vi "Analog Output User Interface.vi"() -> ()   [LabVIEW 2023, in "GUI.lvlib" / "Diagnostic.lvlib"]
uses:
  Diagnostic.lvlib
  Control/Analog Output 6739.ctl
  Control/Analog Output.ctl
  Control/Analog Output 6738.ctl
  HardwareAbstractionLayer_LVOOP/Analog Output/NI Analog Output/NI Analog Output.lvclass
  D:/eDCU LTT/VT LTT Project/Source Code/HardwareAbstractionLayer_LVOOP/Analog Output/AO/AO.lvclass
  HardwareAbstractionLayer_LVOOP/Database/SQL Public VI/Control/DB Options.ctl
  HardwareAbstractionLayer_LVOOP/Main/Class Ref.ctl
  HardwareAbstractionLayer_LVOOP/DMM/DMM.lvclass
  HardwareAbstractionLayer_LVOOP/Function Generator/Function Generator.lvclass
  HardwareAbstractionLayer_LVOOP/Oscilloscope/Oscilloscope.lvclass
  HardwareAbstractionLayer_LVOOP/PowerSupply/PowerSupply.lvclass
  HardwareAbstractionLayer_LVOOP/Teststand/Teststand.lvclass
  HardwareAbstractionLayer_LVOOP/Analog Output/AO/AO.lvclass
  HardwareAbstractionLayer_LVOOP/Analog Input/AI/AI.lvclass
  HardwareAbstractionLayer_LVOOP/Database/Database.lvclass
  HardwareAbstractionLayer_LVOOP/Digital Output/DO_class/DO.lvclass
  HardwareAbstractionLayer_LVOOP/Digital Input/DI_class/DI.lvclass
  HardwareAbstractionLayer_LVOOP/PWM Output/PWM Output_class/PWM Output.lvclass
  HardwareAbstractionLayer_LVOOP/PWM Input/PWM Input_class/PWM Input.lvclass
  HardwareAbstractionLayer_LVOOP/NI Switch/NISwitch_class/NISwitch.lvclass
  HardwareAbstractionLayer_LVOOP/Modbus/Modbus_class/Modbus.lvclass
  HardwareAbstractionLayer_LVOOP/CAN/CAN Lib/CAN_class/CAN.lvclass
  HardwareAbstractionLayer_LVOOP/Main/Main.lvclass
panel:
  in  "Stop Acquire":bool
  in  "Start Acquire":bool
  out "error out":errorcluster
  in  "error in":errorcluster
  in  "Operation":T1(tab)
  in  "PXIe - 6739 M1":T2 {"Channel 63" min=-10.0 max=10.0 step=0.1 format="%#.2g"; "Channel 62" min=-10.0 max=10.0 step=0.1 format="%#.2g"; "Channel 61" min=-10.0 max=10.0 step=0.1 format="%#.2g"; "Channel 60" min=-10.0 max=10.0 step=0.1 format="%#.2g"; "Channel 59" min=-10.0 max=10.0 step=0.1 format="%#.2g"; "Channel 58" min=-10.0 max=10.0 step=0.1 format="%#.2g"; "Channel 57" min=-10.0 max=10.0 step=0.1 format="%#.2g"; "Channel 56" min=-10.0 max=10.0 step=0.1 format="%#.2g"; "Channel 55" min=-10.0 max=10.0 step=0.1 format="%#.2g"; "Channel 54" min=-10.0 max=10.0 step=0.1 format="%#.2g"; "Channel 53" min=-10.0 max=10.0 step=0.1 format="%#.2g"; "Channel 52" min=-10.0 max=10.0 step=0.1 format="%#.2g"; "Channel 51" min=-10.0 max=10.0 step=0.1 format="%#.2g"; "Channel 50" min=-10.0 max=10.0 step=0.1 format="%#.2g"; "Channel 49" min=-10.0 max=10.0 step=0.1 format="%#.2g"; "Channel 48" min=-10.0 max=10.0 step=0.1 format="%#.2g"; "Channel 47" min=-10.0 max=10.0 step=0.1 format="%#.2g"; "Channel 46" min=-10.0 max=10.0 step=0.1 format="%#.2g"; "Channel 45" min=-10.0 max=10.0 step=0.1 format="%#.2g"; "Channel 44" min=-10.0 max=10.0 step=0.1 format="%#.2g"; "Channel 43" min=-10.0 max=10.0 step=0.1 format="%#.2g"; "Channel 42" min=-10.0 max=10.0 step=0.1 format="%#.2g"; "Channel 41" min=-10.0 max=10.0 step=0.1 format="%#.2g"; "Channel 40" min=-10.0 max=10.0 step=0.1 format="%#.2g"; "Channel 39" min=-10.0 max=10.0 step=0.1 format="%#.2g"; "Channel 38" min=-10.0 max=10.0 step=0.1 format="%#.2g"; "Channel 37" min=-10.0 max=10.0 step=0.1 format="%#.2g"; "Channel 36" min=-10.0 max=10.0 step=0.1 format="%#.2g"; "Channel 35" min=-10.0 max=10.0 step=0.1 format="%#.2g"; "Channel 34" min=-10.0 max=10.0 step=0.1 format="%#.2g"; "Channel 33" min=-10.0 max=10.0 step=0.1 format="%#.2g"; "Channel 32" min=-10.0 max=10.0 step=0.1 format="%#.2g"; "Channel 31" min=-10.0 max=10.0 step=0.1 format="%#.2g"; "Channel 30" min=-10.0 max=10.0 step=0.1 format="%#.2g"; "Channel 29" min=-10.0 max=10.0 step=0.1 format="%#.2g"; "Channel 28" min=-10.0 max=10.0 step=0.1 format="%#.2g"; "Channel 27" min=-10.0 max=10.0 step=0.1 format="%#.2g"; "Channel 26" min=-10.0 max=10.0 step=0.1 format="%#.2g"; "Channel 25" min=-10.0 max=10.0 step=0.1 format="%#.2g"; "Channel 24" min=-10.0 max=10.0 step=0.1 format="%#.2g"; "Channel 23" min=-10.0 max=10.0 step=0.1 format="%#.2g"; "Channel 22" min=-10.0 max=10.0 step=0.1 format="%#.2g"; "Channel 21" min=-10.0 max=10.0 step=0.1 format="%#.2g"; "Channel 20" min=-10.0 max=10.0 step=0.1 format="%#.2g"; "Channel 19" min=-10.0 max=10.0 step=0.1 format="%#.2g"; "Channel 18" min=-10.0 max=10.0 step=0.1 format="%#.2g"; "Channel 17" min=-10.0 max=10.0 step=0.1 format="%#.2g"; "Channel 16" min=-10.0 max=10.0 step=0.1 format="%#.2g"; "Channel 15" min=-10.0 max=10.0 step=0.1 format="%#.2g"; "Channel 14" min=-10.0 max=10.0 step=0.1 format="%#.2g"; "Channel 13" min=-10.0 max=10.0 step=0.1 format="%#.2g"; "Channel 12" min=-10.0 max=10.0 step=0.1 format="%#.2g"; "Channel 11" min=-10.0 max=10.0 step=0.1 format="%#.2g"; "Channel 10" min=-10.0 max=10.0 step=0.1 format="%#.2g"; "Channel 9" min=-10.0 max=10.0 step=0.1 format="%#.2g"; "Channel 8" min=-10.0 max=10.0 step=0.1 format="%#.2g"; "Channel 7" min=-10.0 max=10.0 step=0.1 format="%#.2g"; "Channel 6" min=-10.0 max=10.0 step=0.1 format="%#.2g"; "Channel 5" min=-10.0 max=10.0 step=0.1 format="%#.2g"; "Channel 4" min=-10.0 max=10.0 step=0.1 format="%#.2g"; "Channel 3" min=-10.0 max=10.0 step=0.1 format="%#.2g"; "Channel 2" min=-10.0 max=10.0 step=0.1 format="%#.2g"; "Channel 1" min=-10.0 max=10.0 step=0.1 format="%#.2g"; "Channel 0" min=-10.0 max=10.0 step=0.1 format="%#.2g"}
  in  "PXIe - 6739 M2":T2 {"Channel 63" min=-10.0 max=10.0 step=0.1 format="%#.2g"; "Channel 62" min=-10.0 max=10.0 step=0.1 format="%#.2g"; "Channel 61" min=-10.0 max=10.0 step=0.1 format="%#.2g"; "Channel 60" min=-10.0 max=10.0 step=0.1 format="%#.2g"; "Channel 59" min=-10.0 max=10.0 step=0.1 format="%#.2g"; "Channel 58" min=-10.0 max=10.0 step=0.1 format="%#.2g"; "Channel 57" min=-10.0 max=10.0 step=0.1 format="%#.2g"; "Channel 56" min=-10.0 max=10.0 step=0.1 format="%#.2g"; "Channel 55" min=-10.0 max=10.0 step=0.1 format="%#.2g"; "Channel 54" min=-10.0 max=10.0 step=0.1 format="%#.2g"; "Channel 53" min=-10.0 max=10.0 step=0.1 format="%#.2g"; "Channel 52" min=-10.0 max=10.0 step=0.1 format="%#.2g"; "Channel 51" min=-10.0 max=10.0 step=0.1 format="%#.2g"; "Channel 50" min=-10.0 max=10.0 step=0.1 format="%#.2g"; "Channel 49" min=-10.0 max=10.0 step=0.1 format="%#.2g"; "Channel 48" min=-10.0 max=10.0 step=0.1 format="%#.2g"; "Channel 47" min=-10.0 max=10.0 step=0.1 format="%#.2g"; "Channel 46" min=-10.0 max=10.0 step=0.1 format="%#.2g"; "Channel 45" min=-10.0 max=10.0 step=0.1 format="%#.2g"; "Channel 44" min=-10.0 max=10.0 step=0.1 format="%#.2g"; "Channel 43" min=-10.0 max=10.0 step=0.1 format="%#.2g"; "Channel 42" min=-10.0 max=10.0 step=0.1 format="%#.2g"; "Channel 41" min=-10.0 max=10.0 step=0.1 format="%#.2g"; "Channel 40" min=-10.0 max=10.0 step=0.1 format="%#.2g"; "Channel 39" min=-10.0 max=10.0 step=0.1 format="%#.2g"; "Channel 38" min=-10.0 max=10.0 step=0.1 format="%#.2g"; "Channel 37" min=-10.0 max=10.0 step=0.1 format="%#.2g"; "Channel 36" min=-10.0 max=10.0 step=0.1 format="%#.2g"; "Channel 35" min=-10.0 max=10.0 step=0.1 format="%#.2g"; "Channel 34" min=-10.0 max=10.0 step=0.1 format="%#.2g"; "Channel 33" min=-10.0 max=10.0 step=0.1 format="%#.2g"; "Channel 32" min=-10.0 max=10.0 step=0.1 format="%#.2g"; "Channel 31" min=-10.0 max=10.0 step=0.1 format="%#.2g"; "Channel 30" min=-10.0 max=10.0 step=0.1 format="%#.2g"; "Channel 29" min=-10.0 max=10.0 step=0.1 format="%#.2g"; "Channel 28" min=-10.0 max=10.0 step=0.1 format="%#.2g"; "Channel 27" min=-10.0 max=10.0 step=0.1 format="%#.2g"; "Channel 26" min=-10.0 max=10.0 step=0.1 format="%#.2g"; "Channel 25" min=-10.0 max=10.0 step=0.1 format="%#.2g"; "Channel 24" min=-10.0 max=10.0 step=0.1 format="%#.2g"; "Channel 23" min=-10.0 max=10.0 step=0.1 format="%#.2g"; "Channel 22" min=-10.0 max=10.0 step=0.1 format="%#.2g"; "Channel 21" min=-10.0 max=10.0 step=0.1 format="%#.2g"; "Channel 20" min=-10.0 max=10.0 step=0.1 format="%#.2g"; "Channel 19" min=-10.0 max=10.0 step=0.1 format="%#.2g"; "Channel 18" min=-10.0 max=10.0 step=0.1 format="%#.2g"; "Channel 17" min=-10.0 max=10.0 step=0.1 format="%#.2g"; "Channel 16" min=-10.0 max=10.0 step=0.1 format="%#.2g"; "Channel 15" min=-10.0 max=10.0 step=0.1 format="%#.2g"; "Channel 14" min=-10.0 max=10.0 step=0.1 format="%#.2g"; "Channel 13" min=-10.0 max=10.0 step=0.1 format="%#.2g"; "Channel 12" min=-10.0 max=10.0 step=0.1 format="%#.2g"; "Channel 11" min=-10.0 max=10.0 step=0.1 format="%#.2g"; "Channel 10" min=-10.0 max=10.0 step=0.1 format="%#.2g"; "Channel 9" min=-10.0 max=10.0 step=0.1 format="%#.2g"; "Channel 8" min=-10.0 max=10.0 step=0.1 format="%#.2g"; "Channel 7" min=-10.0 max=10.0 step=0.1 format="%#.2g"; "Channel 6" min=-10.0 max=10.0 step=0.1 format="%#.2g"; "Channel 5" min=-10.0 max=10.0 step=0.1 format="%#.2g"; "Channel 4" min=-10.0 max=10.0 step=0.1 format="%#.2g"; "Channel 3" min=-10.0 max=10.0 step=0.1 format="%#.2g"; "Channel 2" min=-10.0 max=10.0 step=0.1 format="%#.2g"; "Channel 1" min=-10.0 max=10.0 step=0.1 format="%#.2g"; "Channel 0" min=-10.0 max=10.0 step=0.1 format="%#.2g"}
  in  "PXIe - 6738 M1":T4 {"Channel 31" min=-10.0 max=10.0 step=0.1 format="%#.2g"; "Channel 30" min=-10.0 max=10.0 step=0.1 format="%#.2g"; "Channel 29" min=-10.0 max=10.0 step=0.1 format="%#.2g"; "Channel 28" min=-10.0 max=10.0 step=0.1 format="%#.2g"; "Channel 27" min=-10.0 max=10.0 step=0.1 format="%#.2g"; "Channel 26" min=-10.0 max=10.0 step=0.1 format="%#.2g"; "Channel 25" min=-10.0 max=10.0 step=0.1 format="%#.2g"; "Channel 24" min=-10.0 max=10.0 step=0.1 format="%#.2g"; "Channel 23" min=-10.0 max=10.0 step=0.1 format="%#.2g"; "Channel 22" min=-10.0 max=10.0 step=0.1 format="%#.2g"; "Channel 21" min=-10.0 max=10.0 step=0.1 format="%#.2g"; "Channel 20" min=-10.0 max=10.0 step=0.1 format="%#.2g"; "Channel 19" min=-10.0 max=10.0 step=0.1 format="%#.2g"; "Channel 18" min=-10.0 max=10.0 step=0.1 format="%#.2g"; "Channel 17" min=-10.0 max=10.0 step=0.1 format="%#.2g"; "Channel 16" min=-10.0 max=10.0 step=0.1 format="%#.2g"; "Channel 15" min=-10.0 max=10.0 step=0.1 format="%#.2g"; "Channel 14" min=-10.0 max=10.0 step=0.1 format="%#.2g"; "Channel 13" min=-10.0 max=10.0 step=0.1 format="%#.2g"; "Channel 12" min=-10.0 max=10.0 step=0.1 format="%#.2g"; "Channel 11" min=-10.0 max=10.0 step=0.1 format="%#.2g"; "Channel 10" min=-10.0 max=10.0 step=0.1 format="%#.2g"; "Channel 9" min=-10.0 max=10.0 step=0.1 format="%#.2g"; "Channel 8" min=-10.0 max=10.0 step=0.1 format="%#.2g"; "Channel 7" min=-10.0 max=10.0 step=0.1 format="%#.2g"; "Channel 6" min=-10.0 max=10.0 step=0.1 format="%#.2g"; "Channel 5" min=-10.0 max=10.0 step=0.1 format="%#.2g"; "Channel 4" min=-10.0 max=10.0 step=0.1 format="%#.2g"; "Channel 3" min=-10.0 max=10.0 step=0.1 format="%#.2g"; "Channel 2" min=-10.0 max=10.0 step=0.1 format="%#.2g"; "Channel 1" min=-10.0 max=10.0 step=0.1 format="%#.2g"; "Channel 0" min=-10.0 max=10.0 step=0.1 format="%#.2g"}
  in  "Stop":bool caption="Blank"
  in  "Write":bool caption="Blank"
  # "Analog Output"
  # "Device:"
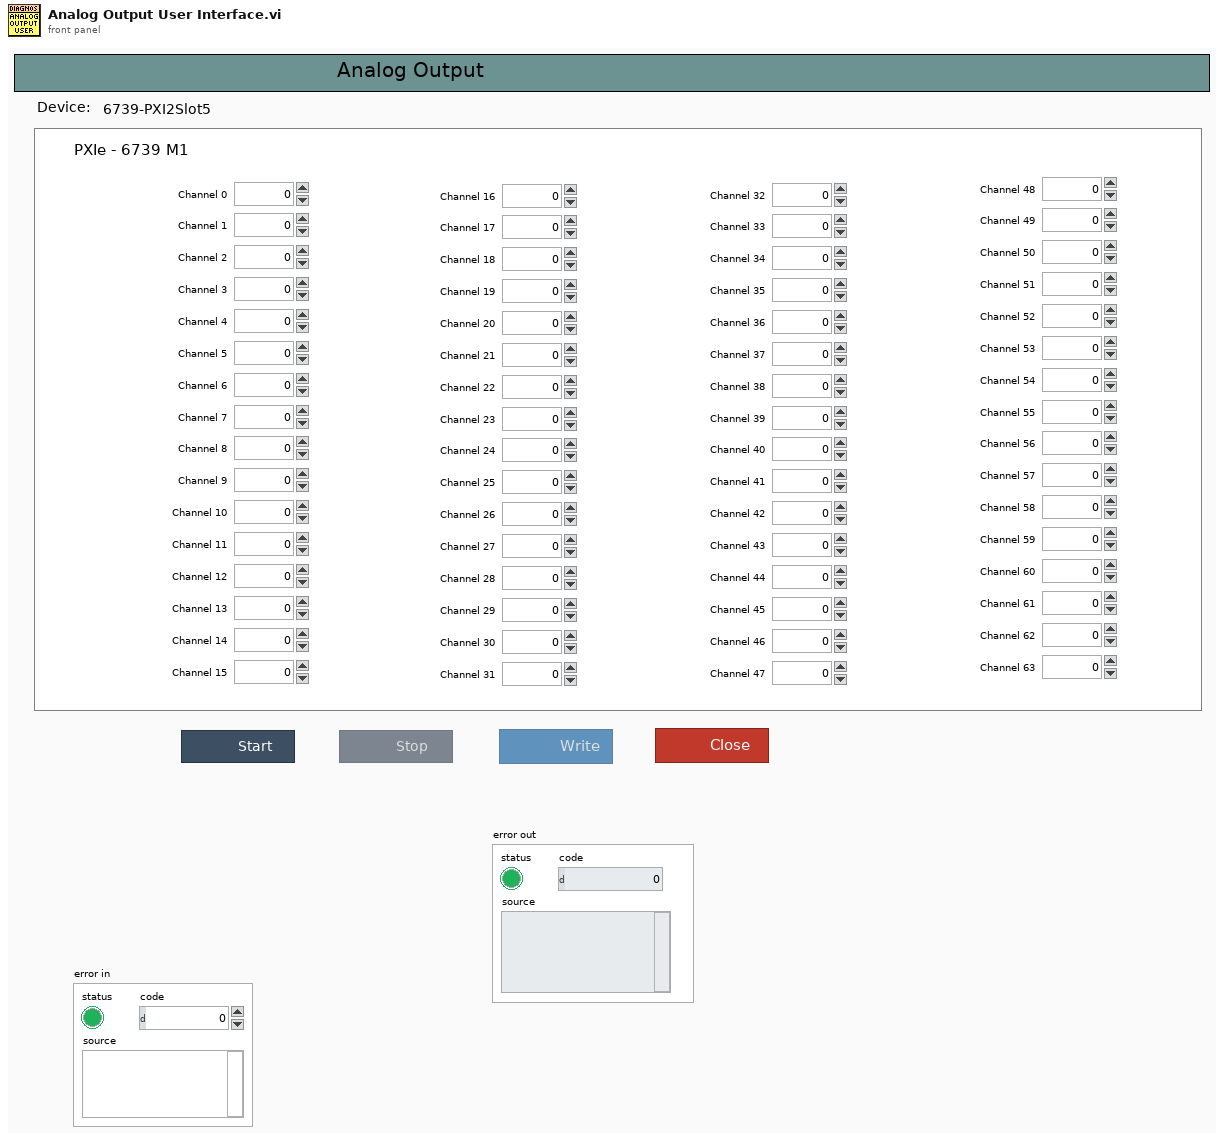
[diagram p1: front panel]
types:
  T1 = enum32{"6739-PXI2Slot5", "6739-PXI2Slot6", "6738-PXI2Slot4"}
  T2 = typedef "GUI.lvlib/Diagnostic.lvlib/Analog Output 6739.ctl" = cluster{"Channel 0":T3, "Channel 1":T3, "Channel 2":T3, "Channel 3":T3, "Channel 4":T3, "Channel 5":T3, "Channel 6":T3, "Channel 7":T3, "Channel 8":T3, "Channel 9":T3, "Channel 10":T3, "Channel 11":T3, "Channel 12":T3, "Channel 13":T3, "Channel 14":T3, "Channel 15":T3, "Channel 16":T3, "Channel 17":T3, "Channel 18":T3, "Channel 19":T3, "Channel 20":T3, "Channel 21":T3, "Channel 22":T3, "Channel 23":T3, "Channel 24":T3, "Channel 25":T3, "Channel 26":T3, "Channel 27":T3, "Channel 28":T3, "Channel 29":T3, "Channel 30":T3, "Channel 31":T3, "Channel 32":T3, "Channel 33":T3, "Channel 34":T3, "Channel 35":T3, "Channel 36":T3, "Channel 37":T3, "Channel 38":T3, "Channel 39":T3, "Channel 40":T3, "Channel 41":T3, "Channel 42":T3, "Channel 43":T3, "Channel 44":T3, "Channel 45":T3, "Channel 46":T3, "Channel 47":T3, "Channel 48":T3, "Channel 49":T3, "Channel 50":T3, "Channel 51":T3, "Channel 52":T3, "Channel 53":T3, "Channel 54":T3, "Channel 55":T3, "Channel 56":T3, "Channel 57":T3, "Channel 58":T3, "Channel 59":T3, "Channel 60":T3, "Channel 61":T3, "Channel 62":T3, "Channel 63":T3}
  T3 = typedef "GUI.lvlib/Diagnostic.lvlib/Analog Output.ctl" = dbl
  T4 = typedef "GUI.lvlib/Diagnostic.lvlib/Analog Output 6738.ctl" = cluster{"Channel 0":T3, "Channel 1":T3, "Channel 2":T3, "Channel 3":T3, "Channel 4":T3, "Channel 5":T3, "Channel 6":T3, "Channel 7":T3, "Channel 8":T3, "Channel 9":T3, "Channel 10":T3, "Channel 11":T3, "Channel 12":T3, "Channel 13":T3, "Channel 14":T3, "Channel 15":T3, "Channel 16":T3, "Channel 17":T3, "Channel 18":T3, "Channel 19":T3, "Channel 20":T3, "Channel 21":T3, "Channel 22":T3, "Channel 23":T3, "Channel 24":T3, "Channel 25":T3, "Channel 26":T3, "Channel 27":T3, "Channel 28":T3, "Channel 29":T3, "Channel 30":T3, "Channel 31":T3}
  T5 = typedef "HardwareAbstractionLayer_LVOOP.lvlib/Database.lvclass/DB Options.ctl" = enum16{"Init", "Select Data", "Insert Data", "Update Data", "Delete Data", "Execute Query", "Create Schema", "Create Table", "List Tables", "List Columns", "Close"}
  T6 = typedef "HardwareAbstractionLayer_LVOOP.lvlib/Main.lvclass/Class Ref.ctl" = cluster{"DMM":refnum<class "DMM.lvclass">, "Function Generator":refnum<class "Function Generator.lvclass">, "Oscilloscope":refnum<class "Oscilloscope.lvclass">, "PowerSupply":refnum<class "PowerSupply.lvclass">, "Teststand":refnum<class "Teststand.lvclass">, "AO":refnum<class "AO.lvclass">, "AI":refnum<class "AI.lvclass">, "Database":refnum<class "Database.lvclass">, "AO Waveform Generation":refnum<class "AO.lvclass">, "DO":refnum<class "DO.lvclass">, "DI":refnum<class "DI.lvclass">, "PWM Output":refnum<class "PWM Output.lvclass">, "PWM Input":refnum<class "PWM Input.lvclass">, "RelayOutput":refnum<class "NISwitch.lvclass">, "Modbus":refnum<class "Modbus.lvclass">, "CAN":refnum<class "CAN.lvclass">}
  T7 = enum8{"Enabled", "Disabled", "Disabled and Grayed Out"}
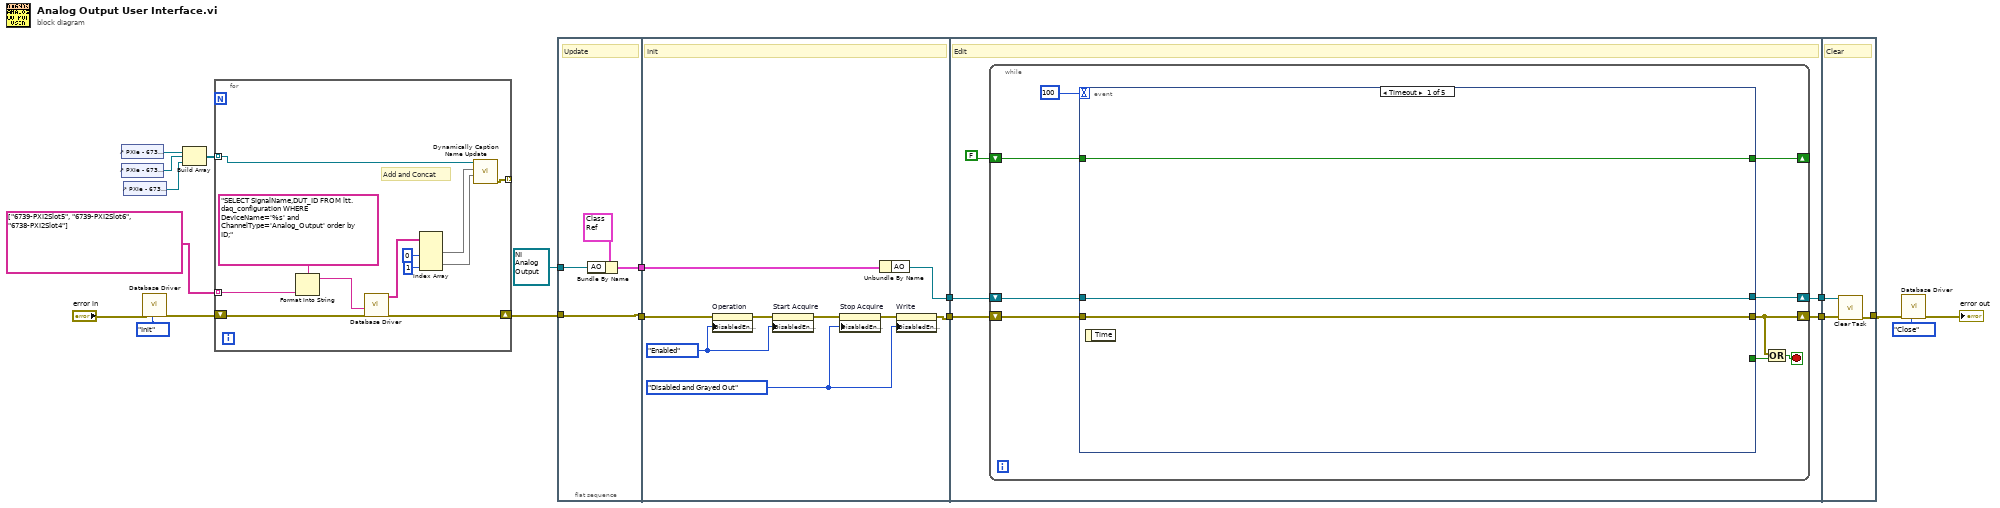
[diagram p0: block diagram]
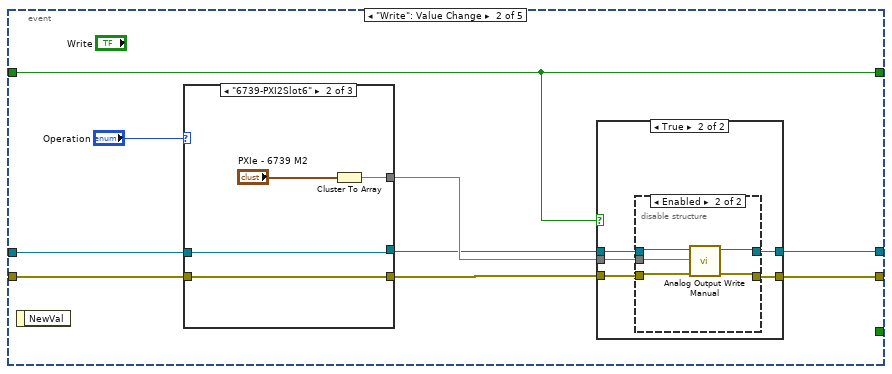
[diagram p2: hidden frame]
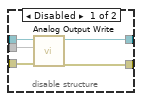
[diagram p4: hidden frame]
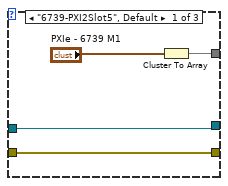
[diagram p5: hidden frame]
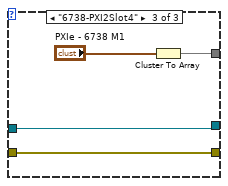
[diagram p6: hidden frame]
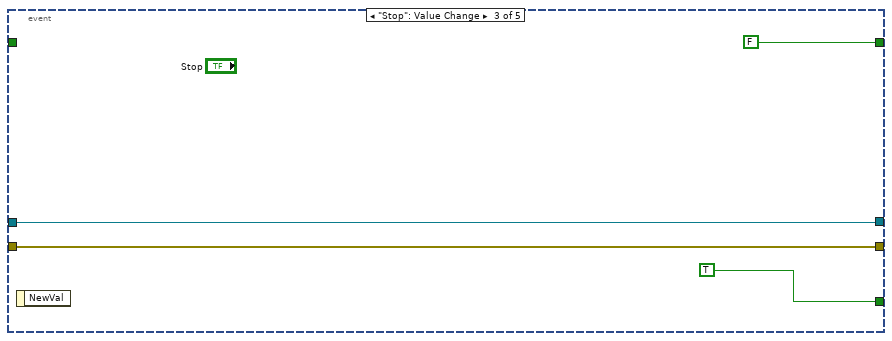
[diagram p7: hidden frame]
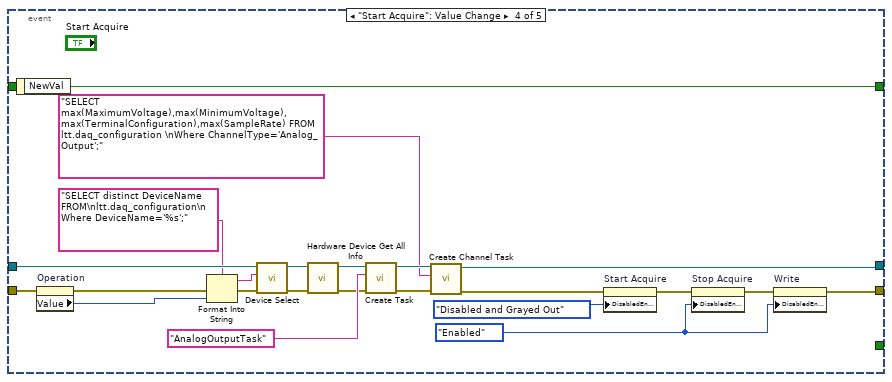
[diagram p8: hidden frame]
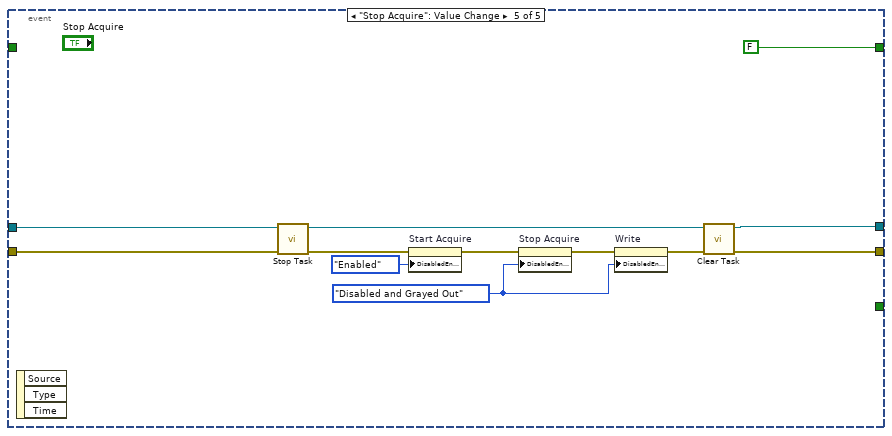
[diagram p9: hidden frame]
diagram:
  n1 = control-ref of="PXIe - 6739 M1"() -> (w5:refnum<vi>)
  n2 = control-ref of="PXIe - 6739 M2"() -> (w4:refnum<vi>)
  n3 = control-ref of="PXIe - 6738 M1"() -> (w3:refnum<vi>)
  n4 = call "Database Driver.vi"("Options"=DB_Options."Init", "error in"="error in") -> ("error out"=w7:errorcluster)  [unwired: 6 in, 3 out]
  n5 = Build Array(w5, w4, w3) -> (w2:refnum<vi>[])
  n6 = for {
    shift-right: [w30] -> w6
    shift-left: w7 -> [w31]
    tunnel: w2 -> [w24] mode=indexing
    tunnel: string[] ["6739-PXI2Slot5", "6739-PXI2Slot6", "6738-PXI2Slot4"] -> [w23] mode=indexing
    tunnel: [w22] -> _ mode=indexing
    # "Add and Concat"
    n7 = Format Into String(format string="SELECT SignalName,DUT_ID FROM ltt.daq_configuration WHERE DeviceName='%s' and ChannelType='Analog_Output' order by ID;", w23) -> (resulting string=w29:string)  [unwired: 2 in, 1 out]
    n8 = call "Database Driver.vi"("error in"=w31, "SQL query"=w29) -> ("error out"=w30:errorcluster, "data"=w27:string[][])  [unwired: 6 in, 2 out]
    n9 = Index Array(array=w27, index (col) #1=0 ("disabled index (col)"), index (col) #2=1 ("index (col)")) -> (element #1=w25:string[], element #2=w20:string[])  [unwired: 2 in]
    n10 = call "Dynamically Caption Name Update.vi"("DUT_Number"=w20, "Caption Name"=w25, "Clust Refnum"=w24) -> ("error out"=w22:errorcluster)  [unwired: 8 in]
  }
  n11 = flat-sequence {
    tunnel: [w32] -> w19
    tunnel: refnum<class "NI Analog Output.lvclass"> refnum ("HardwareAbstractionLayer_LVOOP.lvlib:NI Analog Output.lvclass") -> [w34]
    tunnel: [w33] -> w16
    tunnel: w6 -> [w32]
    tunnel: w19 -> [w41]
    tunnel: [w37] -> w18
    tunnel: w16 -> [w44]
    tunnel: [w43] -> w15
    tunnel: w18 -> [w49]
    tunnel: w15 -> [w48]
    tunnel: [w47] -> w14
    tunnel: [w46] -> w13
    tunnel: [w139] -> w11
    tunnel: w14 -> [w141]
    tunnel: w13 -> [w140]
    frame #0 {
      # "Update"
      n12 = Bundle By Name(cluster=T6 {"DMM"=refnum, "Function Generator"=refnum, "Oscilloscope"=refnum, "PowerSupply"=refnum, "Teststand"=refnum, "AO"=refnum, "AI"=refnum, "Database"=refnum, "AO Waveform Generation"=refnum, "DO"=refnum, "DI"=refnum, "PWM Output"=refnum, "PWM Input"=refnum, "RelayOutput"=refnum, "Modbus"=refnum, "CAN"=refnum} ("Class Cluster"), "AO"=w34) -> (w33:T6)
    }
    frame #1 {
      w36 = T7."Disabled and Grayed Out" ("Disabled")
      w39 = T7."Enabled" ("Disabled")
      # "Init"
      n13 = property on="Operation" class="TabCtl (strict)"(error in=w41, "DisabledEnum"=w39) -> (error out=w40:errorcluster)  [unwired: 1 in, 1 out]
      n14 = property on="Start Acquire" class="Bool"(error in=w40, "DisabledEnum"=w39) -> (error out=w42:errorcluster)  [unwired: 1 in, 1 out]
      n15 = property on="Stop Acquire" class="Bool"(error in=w42, "DisabledEnum"=w36) -> (error out=w38:errorcluster)  [unwired: 1 in, 1 out]
      n16 = Unbundle By Name(w44) -> ("AO"=w43:refnum<class "AO.lvclass">)
      n17 = property on="Write" class="Bool (strict)"(error in=w38, "DisabledEnum"=w36) -> (error out=w37:errorcluster)  [unwired: 1 in, 1 out]
    }
    frame #2 {
      # "Edit"
      n18 = while {
        shift-right: [w50] -> w47
        shift-left: w49 -> [w55]
        shift-right: [w54] -> w46
        shift-left: w48 -> [w56]
        shift-right: [w53] -> _
        shift-left: FALSE ("NewVal") -> [w52]
        stop <- w51 stop-if-true
        n19 = event shown="[0] Timeout" {
          selector: _ -> [_ _ _ _ _]
          dyn-events: _ -> [_ _ _ _ _]
          timeout: 100 -> [_ _ _ _ _]
          tunnel: [_ _ TRUE ("Stop") _ _] -> w57
          tunnel: w56 -> [w61 w69 w102 w117 w138]
          tunnel: w55 -> [w60 w70 w101 w125 w137]
          tunnel: [w61 w66 w102 w110 w130] -> w54
          tunnel: [w60 w65 w101 w105 w132] -> w50
          tunnel: [w59 w63 FALSE ("NewVal") w126 FALSE ("NewVal")] -> w53
          tunnel: w52 -> [w59 w63 _ _ _]
          event Timeout {
            n20 = event-data() -> ()  [unwired: 1 in, 1 out]
          }
          event "Write": Value Change {
            n21 = event-data() -> ()  [unwired: 1 in, 1 out]
            n22 = case shown="\"6739-PXI2Slot6\"" "Operation" {
              tunnel: w70 -> [w90 w93 w97]
              tunnel: w69 -> [w91 w94 w98]
              tunnel: [w91 w94 w98] -> w62
              tunnel: [w90 w93 w97] -> w67
              tunnel: [w88 w92 w96] -> w64
              frame "6739-PXI2Slot5", Default {
                n23 = Cluster To Array(cluster="PXIe - 6739 M1") -> (array=w88:T3[])
              }
              frame "6739-PXI2Slot6" {
                n24 = Cluster To Array(cluster="PXIe - 6739 M2") -> (array=w92:T3[])
              }
              frame "6738-PXI2Slot4" {
                n25 = Cluster To Array(cluster="PXIe - 6738 M1") -> (array=w96:T3[])
              }
            }
            n26 = case shown="True" w63 {
              tunnel: w62 -> [w72 w77]
              tunnel: w67 -> [w71 w76]
              tunnel: [w72 w75] -> w66
              tunnel: [w71 w74] -> w65
              tunnel: w64 -> [_ w73]
              frame False {
              }
              frame True {
                n27 = disable-structure shown="Enabled" {
                  disable-tunnel: w77 -> [w82 w87]
                  disable-tunnel: w76 -> [w81 w84]
                  disable-tunnel: [w80 w86] -> w75
                  disable-tunnel: [w79 w85] -> w74
                  disable-tunnel: w73 -> [w78 w83]
                  frame Disabled {
                    n28 = call-dynamic "Analog Output Write.vi"("error in (no error)"=w81, "Analog Output Write"=w78, "AO in"=w82) -> ("error out"=w79:errorcluster, "AO out"=w80:refnum<class "AO.lvclass">)  [unwired: 7 in]
                  }
                  frame Enabled {
                    n29 = call-dynamic "Analog Output Write Manual.vi"("error in (no error)"=w84, "Analog Output Write"=w83, "AO in"=w87) -> ("error out"=w85:errorcluster, "AO out"=w86:refnum<class "AO.lvclass">)  [unwired: 7 in]
                  }
                }
              }
            }
          }
          event "Stop": Value Change {
            n30 = event-data() -> ()  [unwired: 1 in, 1 out]
          }
          event "Start Acquire": Value Change {
            w104 = T7."Enabled" ("Disabled")
            n31 = event-data() -> ("NewVal"=w126:bool)  [unwired: 1 in]
            n32 = property on="Operation" class="TabCtl (strict)"(error in=w125) -> (error out=w114:errorcluster, "Value"=w115:T1)  [unwired: 1 in, 1 out]
            n33 = Format Into String(format string="SELECT distinct DeviceName FROM\nltt.daq_configuration\n Where DeviceName='%s';" ("SQL query"), error in=w114, w115) -> (resulting string=w112:string, error out=w113:errorcluster)  [unwired: 1 in]
            n34 = call-dynamic "Device Select.vi"("error in (no error)"=w113, "SQL query"=w112, "AO in"=w117) -> ("error out"=w120:errorcluster, "AO out"=w121:refnum<class "AO.lvclass">)  [unwired: 7 in]
            n35 = call-dynamic "Hardware Device Get All Info.vi"("error in (no error)"=w120, "AO in"=w121) -> ("error out"=w118:errorcluster, "AO out"=w119:refnum<class "AO.lvclass">)  [unwired: 8 in]
            n36 = call-dynamic "Create Task.vi"("error in (no error)"=w118, "Task name"="AnalogOutputTask", "AO in"=w119) -> ("error out"=w124:errorcluster, "AO out"=w123:refnum<class "AO.lvclass">)  [unwired: 7 in]
            n37 = call-dynamic "Create Channel Task.vi"("error in (no error)"=w124, "SQL query"="SELECT max(MaximumVoltage),max(MinimumVoltage), max(TerminalConfiguration),max(SampleRate) FROM ltt.daq_configuration \nWhere ChannelType='Analog_Output';", "AO in"=w123) -> ("error out"=w107:errorcluster, "AO out"=w110:refnum<class "AO.lvclass">)  [unwired: 7 in]
            n38 = property on="Start Acquire" class="Bool"(error in=w107, "DisabledEnum"=T7."Disabled and Grayed Out" ("Disabled")) -> (error out=w109:errorcluster)  [unwired: 1 in, 1 out]
            n39 = property on="Stop Acquire" class="Bool"(error in=w109, "DisabledEnum"=w104) -> (error out=w106:errorcluster)  [unwired: 1 in, 1 out]
            n40 = property on="Write" class="Bool (strict)"(error in=w106, "DisabledEnum"=w104) -> (error out=w105:errorcluster)  [unwired: 1 in, 1 out]
          }
          event "Stop Acquire": Value Change {
            w127 = T7."Disabled and Grayed Out" ("Disabled")
            n41 = event-data() -> ()  [unwired: 1 in, 3 out]
            n42 = call-dynamic "Stop Task.vi"("error in (no error)"=w137, "AO in"=w138) -> ("error out"=w134:errorcluster, "AO out"=w131:refnum<class "AO.lvclass">)  [unwired: 8 in]
            n43 = property on="Start Acquire" class="Bool"(error in=w134, "DisabledEnum"=T7."Enabled" ("Disabled")) -> (error out=w136:errorcluster)  [unwired: 1 in, 1 out]
            n44 = property on="Stop Acquire" class="Bool"(error in=w136, "DisabledEnum"=w127) -> (error out=w129:errorcluster)  [unwired: 1 in, 1 out]
            n45 = property on="Write" class="Bool (strict)"(error in=w129, "DisabledEnum"=w127) -> (error out=w128:errorcluster)  [unwired: 1 in, 1 out]
            n46 = call-dynamic "Clear Task.vi"("error in (no error)"=w128, "AO in"=w131) -> ("error out"=w132:errorcluster, "AO out"=w130:refnum<class "AO.lvclass">)  [unwired: 8 in]
          }
        }
        n47 = Compound Arithmetic op=OR(w50, w57) -> (w51:bool)
      }
    }
    frame #3 {
      # "Clear"
      n48 = call-dynamic "Clear Task.vi"("error in (no error)"=w141, "AO in"=w140) -> ("error out"=w139:errorcluster)  [unwired: 8 in, 1 out]
    }
  }
  n49 = call "Database Driver.vi"("Options"=DB_Options."Close", "error in"=w11) -> ("error out"=→"error out":errorcluster)  [unwired: 6 in, 3 out]
